vi "Destroy.vi"(8 "error in (no error)":errorcluster, 11 "EventDaemon in":refnum<class "ErrorHandler.lvclass">) -> (0 "error out":errorcluster)   [LabVIEW 2024, in "ErrorHandler.lvclass"]
doc: "Destroys events and queues of deamon"
uses:
  ErrorHandler.lvclass
  ErrorHandler.lvclass/ErrorHandler.ctl
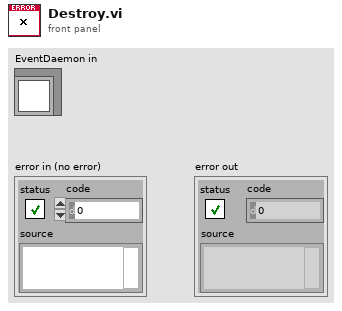
[diagram p1: front panel]
types:
  T1 = typedef "ErrorDaemon.lvclass/msg--cluster.ctl" = cluster{"cmd":T2, "error":errorcluster}
  T2 = typedef "ErrorDaemon.lvclass/states--enum.ctl" = enum16{"init", "default", "display error", "error handler", "exit"}
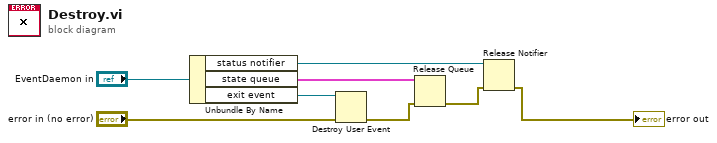
[diagram p0: block diagram]
diagram:
  n1 = Unbundle By Name("EventDaemon in") -> ("status notifier"=w3:refnum<notifier>, "state queue"=w5:T1, "exit event"=w7:refnum<user-event>)
  n2 = Destroy User Event(user event=w7, error in="error in (no error)") -> (error out=w4:errorcluster)
  n3 = Release Queue(queue=w5, error in (no error)=w4) -> (error out=w2:errorcluster)  [unwired: 1 in, 2 out]
  n4 = Release Notifier(notifier=w3, error in (no error)=w2) -> (error out=→"error out":errorcluster)  [unwired: 1 in, 2 out]
